vi "Assert Not Empty Array.vi"(7 "Label":string="Assert Contains", 8 "error in (no error)":errorcluster, 10 "Array":variant[](array[variant])) -> (0 "error out":errorcluster)   [LabVIEW 2017, in "Assert Extensions.lvclass"]
uses:
  Assert Extensions.lvclass
  <vilib>/addons/_JKI Toolkits/Caraya/classes/Properties.Assert/Properties.Assert.lvclass
  C:/Program Files/National Instruments/LabVIEW 2017/vi.lib/addons/_JKI Toolkits/Caraya/classes/Properties/Properties.lvclass
  <vilib>/addons/_JKI Toolkits/Caraya/classes/Assert/Assert.lvclass
  <vilib>/addons/_JKI Toolkits/Caraya/classes/Properties/Properties.lvclass
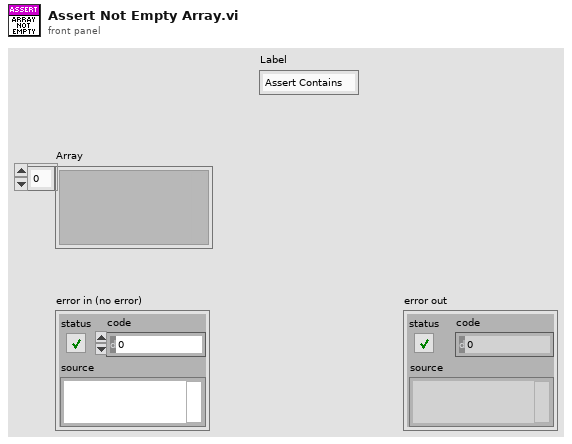
[diagram p1: front panel]
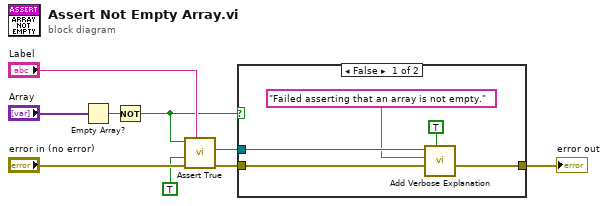
[diagram p0: block diagram]
diagram:
  n1 = Empty Array?(array="Array") -> (empty?=w2:bool)
  n2 = Not(x=w2) -> (.not. x?=w1:bool)
  n3 = call <vilib>:"Assert True.vi"("Label"="Label", "error in (no error)"="error in (no error)", "Register with caller test (F)"=TRUE, "True?"=w1) -> ("error out"=w6:errorcluster, "Properties"=w4:refnum<class "Properties.Assert.lvclass">)  [unwired: 6 in]
  n4 = case shown="False" w1 {
    tunnel: w6 -> [w13 w15]
    tunnel: [w12 w15] -> w5
    tunnel: w4 -> [w11 _]
    frame False {
      n5 = call <vilib>:"Add Verbose Explanation.vi"("overwrite?"=TRUE, "error in (no error)"=w13, "Verbose Explanation"="Failed asserting that an array is not empty.", "Properties"=w11) -> ("error out"=w12:errorcluster)  [unwired: 6 in, 1 out]
    }
    frame True {
    }
  }
  "error out" <- w5
